vi "GUI_SmaractMCS.vi"() -> ()   [LabVIEW 2013]
uses:
  Shared/GUI_Template/GUI_master/tcp_new_data_event.ctl
  Shared/GUI_Template/GUI_master/tcp new data cluster.ctl
panel:
  in  "GUIdevice 1":string
  in  "Tab Control":enum32{"All Channels", "Internal"}(tab)
  in  "Home.Channel 3::1":enum16{"off", "on"}(ring) caption="Home.channel 3"
  in  "Home.Channel 2::1":enum16{"off", "on"}(ring) caption="Home.channel 2"
  in  "Position.Channel 3::1":dbl caption="Position.channel 3" min=0.0 max=10.0
  in  "Position.Channel 2::1":dbl caption="Position.channel 2" min=0.0 max=10.0
  in  "Position.Channel 1::1":dbl caption="Position.channel 1" min=0.0 max=10.0
  in  "Home.Channel 1::1":enum16{"off", "on"}(ring) caption="Home.channel 1"
  in  "localsavingpath::1":path caption="LocalSavingPath"
  out "tcp data event":T1
  in  "Refresh Button":bool
  out "device status::1":string="Initialized" caption="Status"
  in  "STOP":bool
  # "DAQ PAD USER INTERFACE"
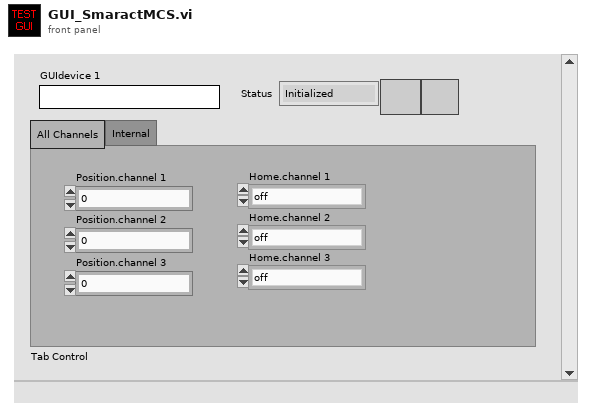
[diagram p1: front panel]
types:
  T1 = typedef "tcp_new_data_event.ctl" = refnum<user-event>
  T2 = enum32{"invalid app kind", "Development System", "Run Time System", "Student Edition", "Embedded LabVIEW", "Evaluation", "Custom"}
  T3 = typedef "tcp new data cluster.ctl" = cluster{"EventEnum":enum16{"new data", "connection status update"}, "Device name":string}
  T4 = enum32{"Invalid", "Standard", "Closed", "Hidden", "Minimized", "Maximized"}
  T5 = cluster{"Core":cluster{"Current VI Reference":refnum<vi>, "Close Panel on Exit?":bool}, "Your Boolean data":bool, "Your string data":string, "SuperGUI":cluster{"STOP queue":refnum<queue>, "SuperGUI ref":refnum<vi>}}
  T6 = cluster{"STOP queue":refnum<queue>, "SuperGUI ref":refnum<vi>}
  T7 = cluster{"Current VI Reference":refnum<vi>, "Close Panel on Exit?":bool}
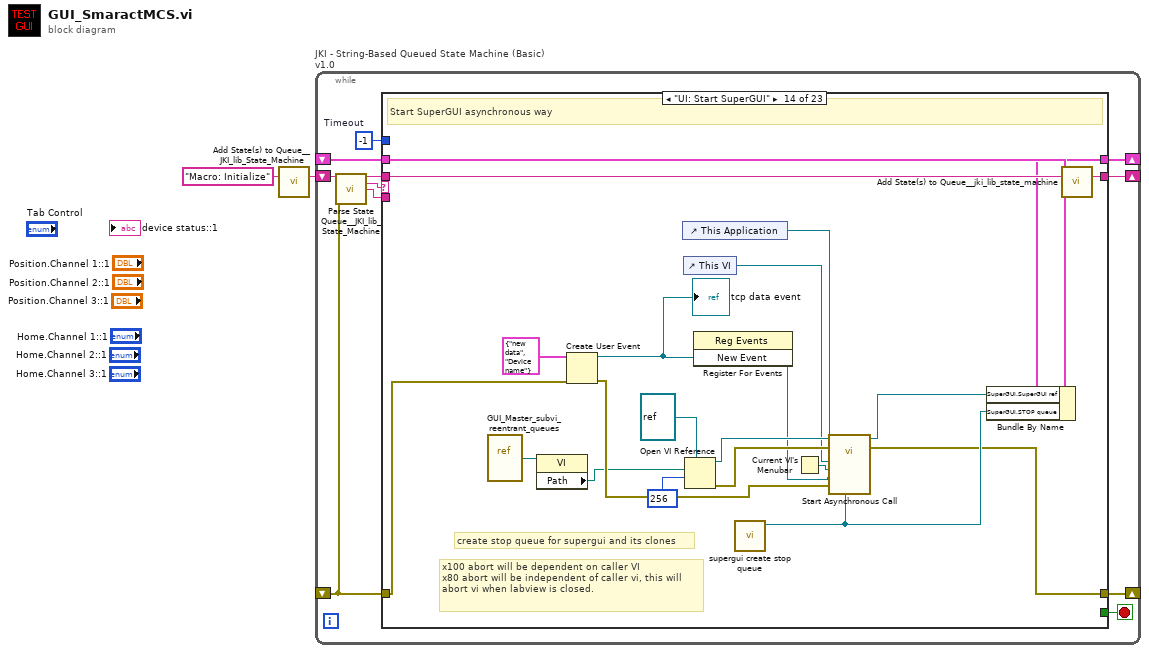
[diagram p0: block diagram]
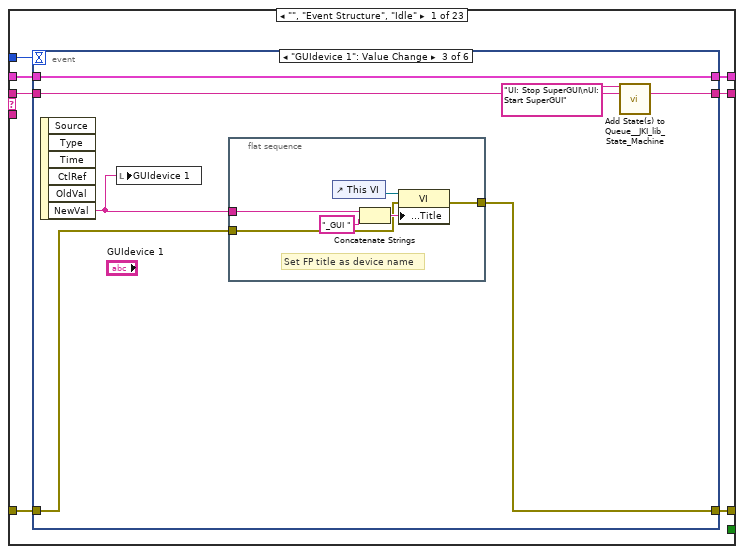
[diagram p2: hidden frame]
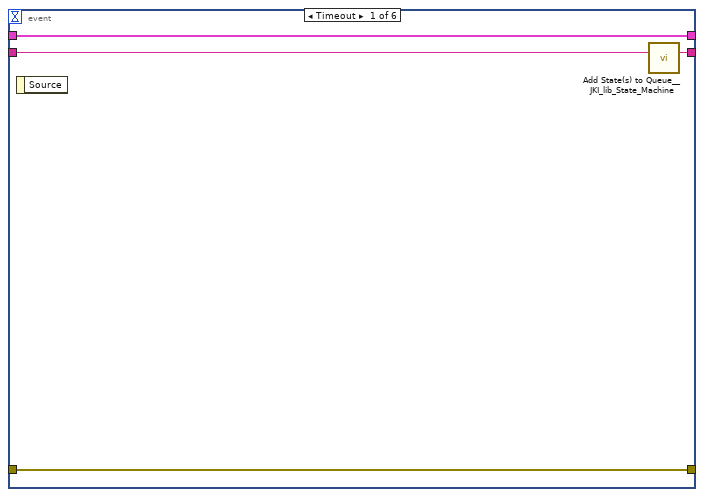
[diagram p3: hidden frame]
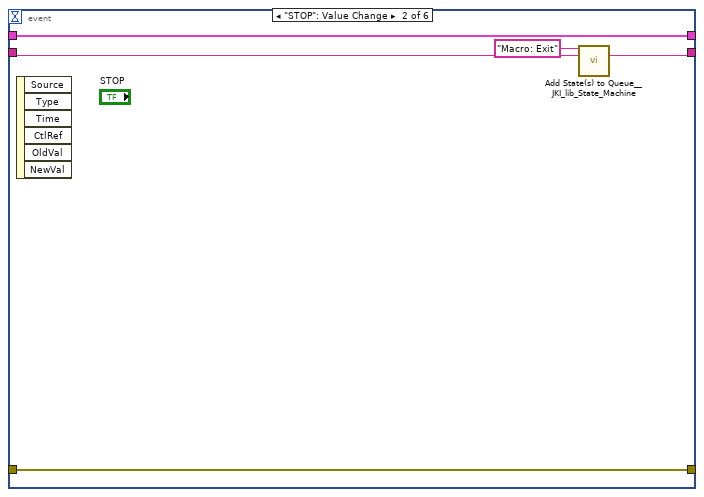
[diagram p4: hidden frame]
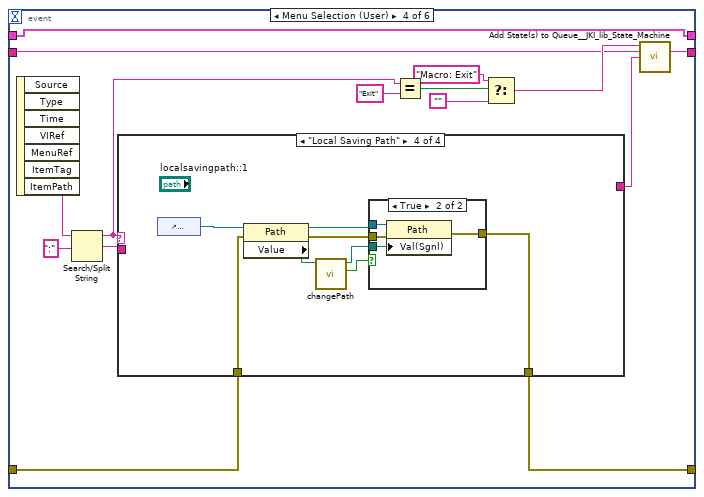
[diagram p5: hidden frame]
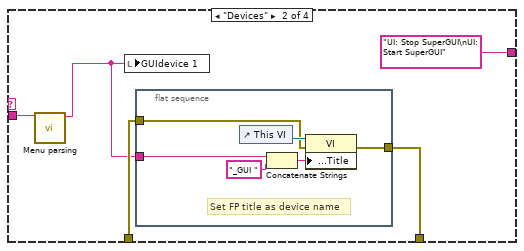
[diagram p7: hidden frame]
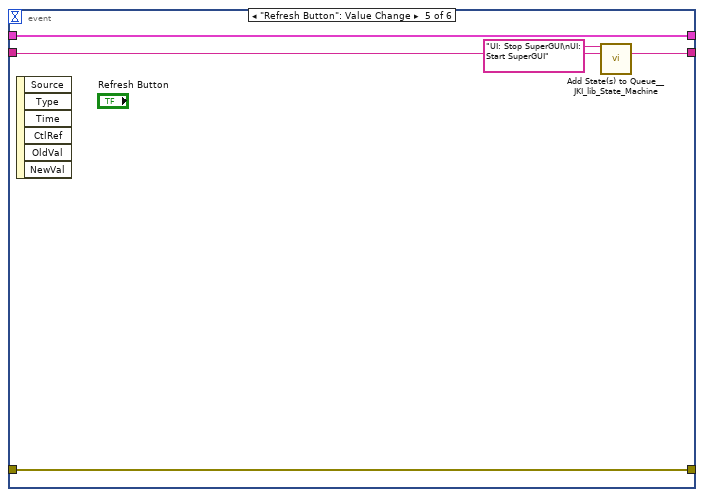
[diagram p10: hidden frame]
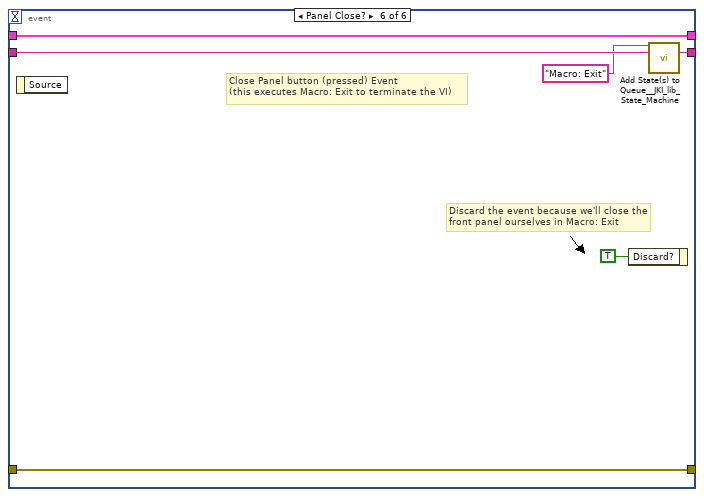
[diagram p11: hidden frame]
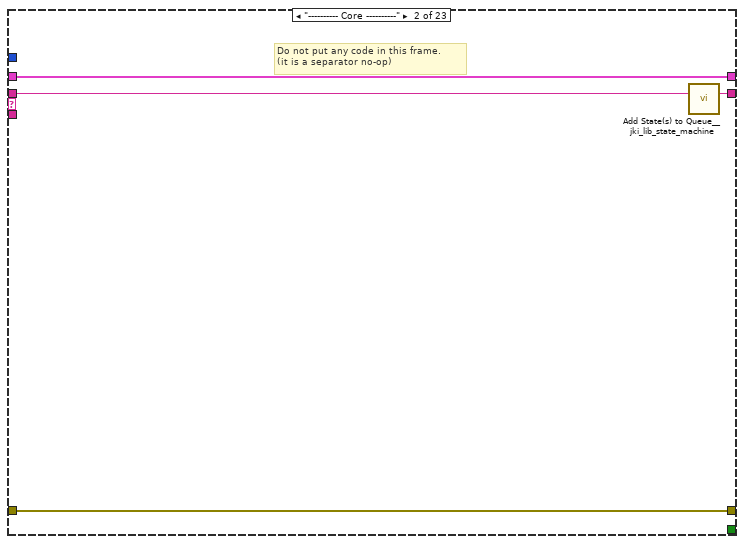
[diagram p12: hidden frame]
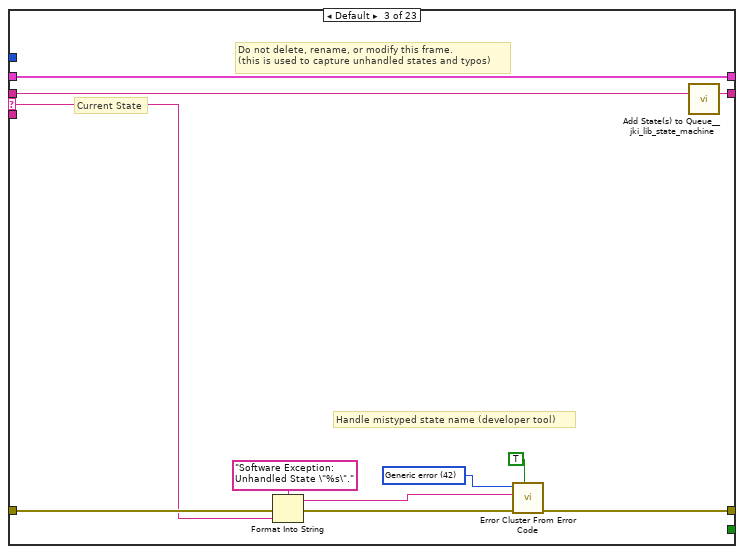
[diagram p13: hidden frame]
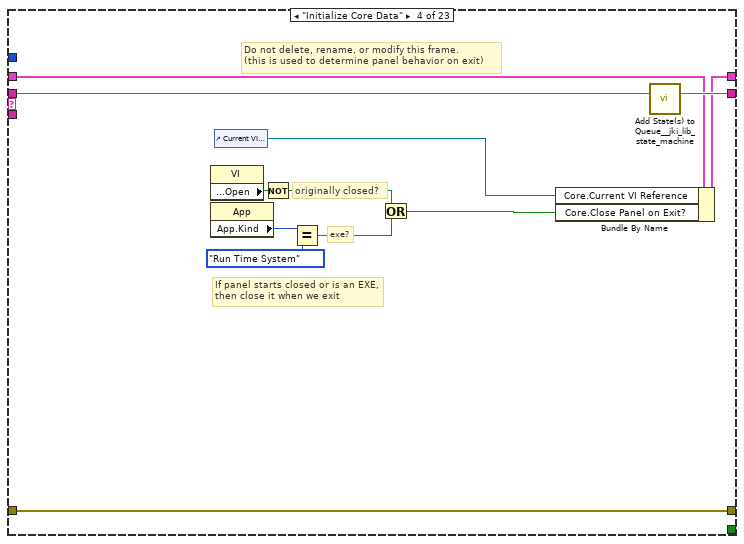
[diagram p14: hidden frame]
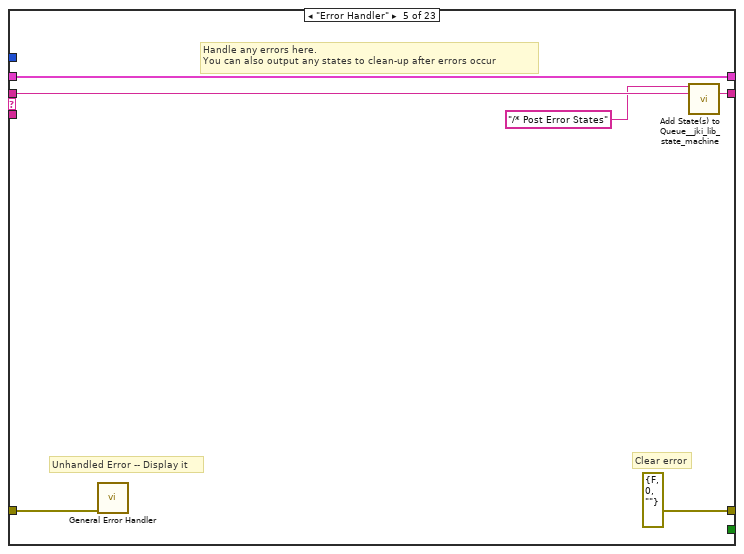
[diagram p15: hidden frame]
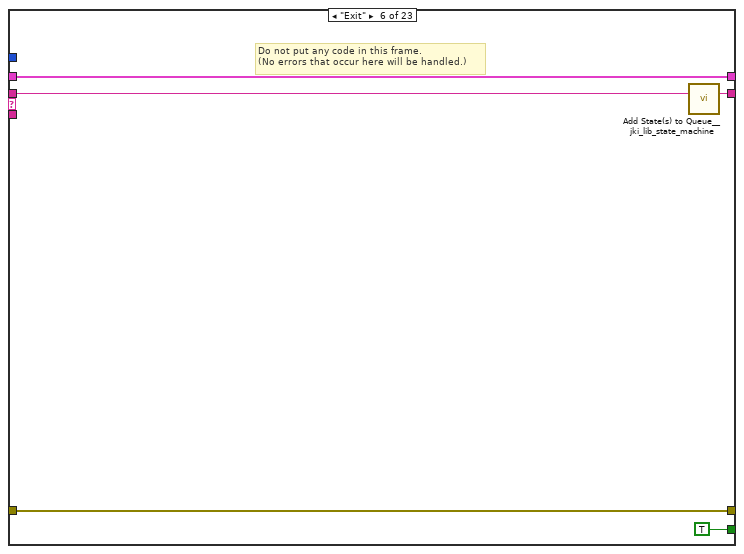
[diagram p16: hidden frame]
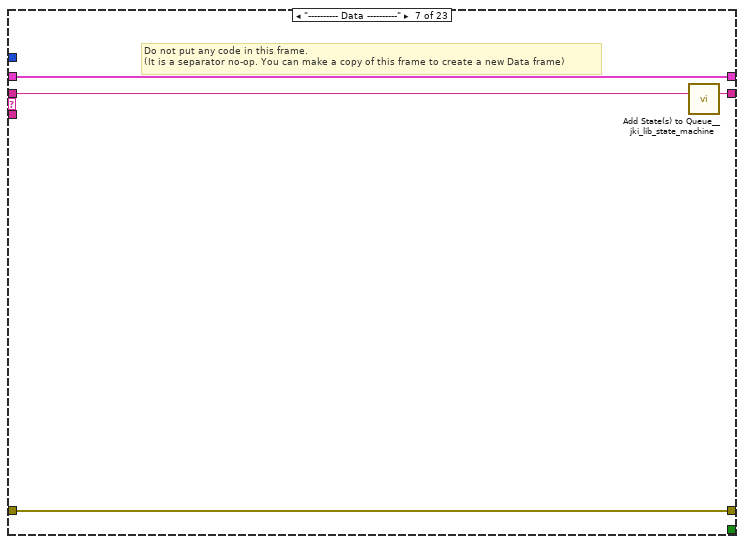
[diagram p17: hidden frame]
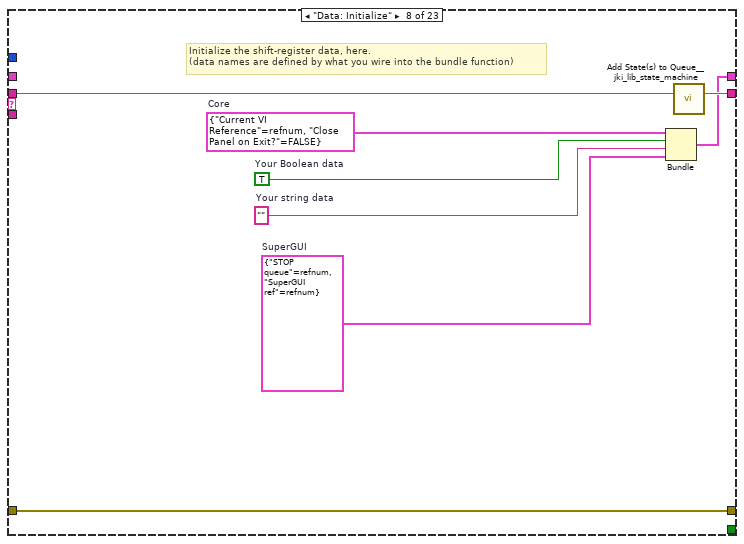
[diagram p18: hidden frame]
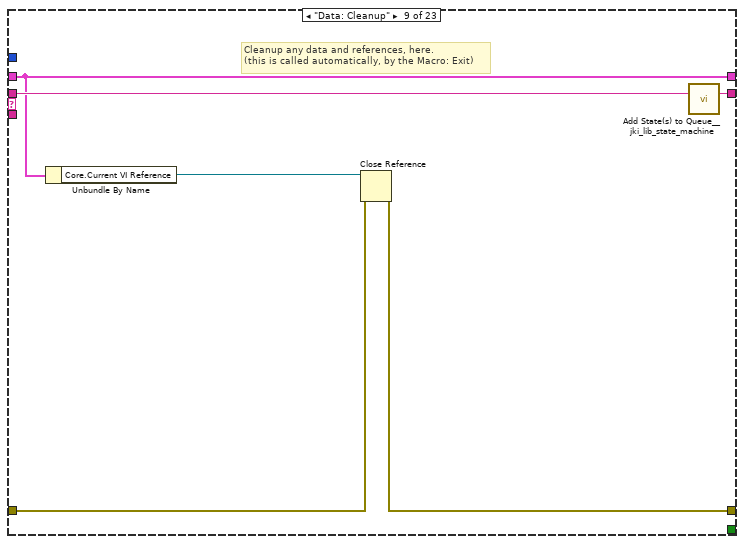
[diagram p19: hidden frame]
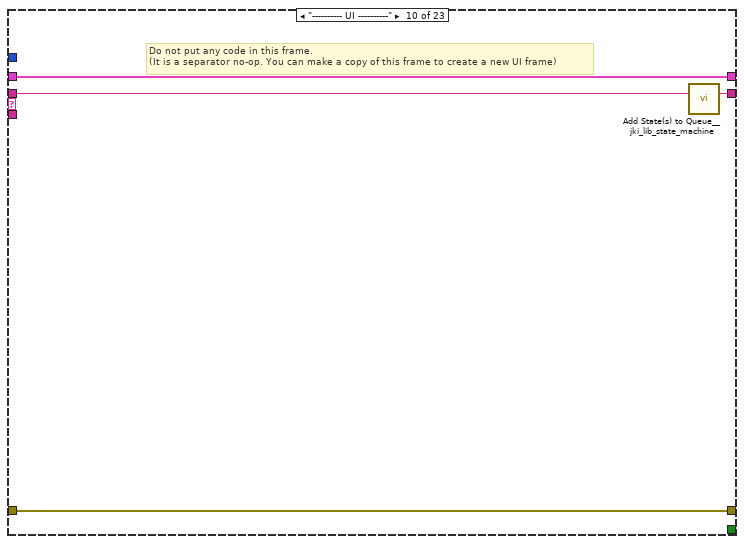
[diagram p20: hidden frame]
diagram:
  n1 = call <vilib>:"Add State(s) to Queue__JKI_lib_State_Machine.vi"("State(s) in (\"\")"="Macro: Initialize") -> ("States Out"=w2:string)  [unwired: 14 in]
  n2 = while "JKI - String-Based Queued State Machine (Basic) v1.0" {
    shift-right: [w6] -> _
    shift-left: _ -> [w5]
    shift-right: [w9] -> _
    shift-left: _ -> [w3]
    shift-right: [w8] -> _
    shift-left: w2 -> [w10]
    stop <- w7 stop-if-true
    w4 = -1  # Timeout
    n3 = call <vilib>:"Parse State Queue__JKI_lib_State_Machine.vi"("State Queue"=w10, "Error In (no error)"=w3) -> ("Remaining States"=w12:string, "Current State"=w13:string, "Arguments"=w11:string)  [unwired: 11 in]
    n4 = case shown="\"UI: Start SuperGUI\"" w13 {
      selector: w13 -> [_ _ w99 _ _ _ _ _ _ _ _ _ _ _ _ _ _ _ _ _ _ _ _]
      tunnel: w12 -> [w20 w98 w103 w121 w127 w132 w136 w144 w150 w154 w158 w166 w198 w232 w240 w246 w257 w283 w288 w298 w302 w306 w310]
      tunnel: w11 -> [_ _ _ _ _ _ _ _ _ _ _ _ _ _ _ w241 w251 _ _ _ _ _ _]
      tunnel: w5 -> [w18 w95 w101 w112 w124 w130 w133 _ w145 w151 w156 w164 w196 w223 w235 w244 w253 w280 w285 w295 w299 w303 w307]
      tunnel: [w17 w96 w105 w118 errorcluster {"status"=FALSE, "code"=0, "source"=""} ("error out") w129 w134 w141 w146 w152 w155 w161 w193 w216 w233 w242 w254 w281 w286 w296 w300 w304 w308] -> w9
      tunnel: w3 -> [w16 w96 w104 w118 w123 w129 w134 w141 w147 w152 w155 w163 w194 w217 w234 w243 w255 w281 w286 w296 w300 w304 w308]
      tunnel: [w19 w97 w102 w120 w126 w131 w135 w143 w149 w153 w157 w165 w197 w231 w239 w245 w256 w282 w287 w297 w301 w305 w309] -> w8
      tunnel: [_ _ _ _ _ TRUE _ _ _ _ _ _ _ _ _ _ _ _ _ _ _ _ _] -> w7
      tunnel: [w15 w95 w101 w119 w124 w130 w133 w142 w145 w151 w156 w164 w196 w222 w235 w244 w253 w280 w285 w295 w299 w303 w307] -> w6
      tunnel: w4 -> [w14 _ _ _ _ _ _ _ _ _ _ _ _ _ _ _ _ _ _ _ _ _ _]
      frame "", "Event Structure", "Idle" {
        n5 = event shown="[2] \"GUIdevice 1\": Value Change" {
          selector: _ -> [_ _ _ _ _ _]
          dyn-events: _ -> [_ _ _ _ _ _]
          timeout: w14 -> [_ _ _ _ _ _]
          tunnel: w20 -> [w24 w27 w33 w51 w86 w94]
          tunnel: [w23 w26 w32 w50 w85 w93] -> w19
          tunnel: w18 -> [w21 w29 w36 w57 w88 w91]
          tunnel: [w22 w28 w34 w44 w87 w92] -> w17
          tunnel: w16 -> [w22 w28 w35 w45 w87 w92]
          tunnel: [w21 w29 w36 w57 w88 w91] -> w15
          event Timeout {
            n6 = event-data() -> ()  [unwired: 1 in, 1 out]
            n7 = call <vilib>:"Add State(s) to Queue__JKI_lib_State_Machine.vi"("State(s) in (\"\")"=w24) -> ("States Out"=w23:string)  [unwired: 14 in]
          }
          event "STOP": Value Change {
            n8 = event-data() -> ()  [unwired: 1 in, 6 out]
            n9 = call <vilib>:"Add State(s) to Queue__JKI_lib_State_Machine.vi"("State(s) in Front (\"\")"="Macro: Exit", "State(s) in (\"\")"=w27) -> ("States Out"=w26:string)  [unwired: 13 in]
          }
          event "GUIdevice 1": Value Change {
            n10 = event-data() -> ("NewVal"=w30:string)  [unwired: 1 in, 5 out]
            n11 = local write "GUIdevice 1"(w30) -> ()
            n12 = flat-sequence {
              tunnel: [w39] -> w34
              tunnel: w35 -> [w38]
              tunnel: w30 -> [w37]
              frame #0 {
                # "Set FP title as device name"
                n13 = control-ref of="This VI"() -> (w42:refnum<vi>)
                n14 = Concatenate Strings(w37, "_GUI ") -> (w41:string)
                n15 = property class="VI"(reference=w42, error in=w38, "Front Panel.Title"=w41) -> (error out=w39:errorcluster)  [unwired: 1 out]
              }
            }
            n16 = call <vilib>:"Add State(s) to Queue__JKI_lib_State_Machine.vi"("State(s) in Front (\"\")"="UI: Stop SuperGUI\nUI: Start SuperGUI", "State(s) in (\"\")"=w33) -> ("States Out"=w32:string)  [unwired: 13 in]
          }
          event Menu Selection (User) {
            n17 = event-data() -> ("ItemPath"=w47:string)  [unwired: 1 in, 6 out]
            n18 = Search/Split String(string=w47, search string/char (-)=":") -> (substring before match=w43:string, match + rest of string=w46:string)  [unwired: 1 in, 1 out]
            n19 = case shown="\"Local Saving Path\"" w43 {
              tunnel: w46 -> [_ w63 _ _]
              tunnel: w45 -> [w58 w62 w70 w73]
              tunnel: [w58 w61 w70 w72] -> w44
              tunnel: [_ "UI: Stop SuperGUI\nUI: Start SuperGUI" _ _] -> w49
              frame "", Default {
              }
              frame "Devices" {
                n20 = call "Menu parsing.vi"("ItemPath"=w63) -> ("ItemPath"=w59:string)  [unwired: 9 in, 1 out]
                n21 = local write "GUIdevice 1"(w59) -> ()
                n22 = flat-sequence {
                  tunnel: [w66] -> w61
                  tunnel: w62 -> [w65]
                  tunnel: w59 -> [w64]
                  frame #0 {
                    # "Set FP title as device name"
                    n23 = control-ref of="This VI"() -> (w69:refnum<vi>)
                    n24 = Concatenate Strings(w64, "_GUI ") -> (w68:string)
                    n25 = property class="VI"(reference=w69, error in=w65, "Front Panel.Title"=w68) -> (error out=w66:errorcluster)  [unwired: 1 out]
                  }
                }
              }
              frame "Exit" {
              }
              frame "Local Saving Path" {
                n26 = control-ref of="localsavingpath::1"() -> (w74:refnum<vi>)
                n27 = property class="Path"(reference=w74, error in=w73) -> (reference out=w76:refnum<vi>, error out=w71:errorcluster, "Value"=w75:path)
                n28 = call "changePath.vi"("Local Saving in (h)"=w75) -> ("change (h)"=w77:bool, "Local Saving out (h)"=w78:path)  [unwired: 9 in]
                n29 = case shown="True" w77 {
                  tunnel: w76 -> [_ w83]
                  tunnel: w78 -> [_ w82]
                  tunnel: [w79 w81] -> w72
                  tunnel: w71 -> [w79 w80]
                  frame False {
                  }
                  frame True {
                    n30 = property class="Path"(reference=w83, error in=w80, "Val(Sgnl)"=w82) -> (error out=w81:errorcluster)  [unwired: 1 out]
                  }
                }
              }
            }
            n31 = Equal?(x=w43, y="Exit") -> (x = y?=w55:bool)
            n32 = Select(t="Macro: Exit", s=w55, f="") -> (s? t:f=w52:string)
            n33 = call <vilib>:"Add State(s) to Queue__JKI_lib_State_Machine.vi"("State(s) in Front (\"\")"=w52, "State(s) in (\"\")"=w51, "State(s) at Back (\"\")"=w49) -> ("States Out"=w50:string)  [unwired: 12 in]
          }
          event "Refresh Button": Value Change {
            n34 = event-data() -> ()  [unwired: 1 in, 6 out]
            n35 = call <vilib>:"Add State(s) to Queue__JKI_lib_State_Machine.vi"("State(s) in Front (\"\")"="UI: Stop SuperGUI\nUI: Start SuperGUI", "State(s) in (\"\")"=w86) -> ("States Out"=w85:string)  [unwired: 13 in]
          }
          event Panel Close? {
            # "Discard the event because we'll close the front panel ourselves in Macro: Exit"
            # "Close Panel button (pressed) Event\n(this executes Macro: Exit to terminate the VI)"
            n36 = event-data() -> ()  [unwired: 1 in, 1 out]
            n37 = event-data("Discard?"=TRUE) -> ()  [unwired: 1 in, 1 out]
            n38 = call <vilib>:"Add State(s) to Queue__JKI_lib_State_Machine.vi"("State(s) in Front (\"\")"="Macro: Exit", "State(s) in (\"\")"=w94) -> ("States Out"=w93:string)  [unwired: 13 in]
          }
        }
      }
      frame "---------- Core ----------" {
        # "Do not put any code in this frame.\n(it is a separator no-op)"
        n39 = call <vilib>:"Add State(s) to Queue__jki_lib_state_machine.vi"("State(s) in (\"\")"=w98) -> ("States Out"=w97:string)  [unwired: 14 in]
      }
      frame Default {
        w108 = 42 items=["No error", "Argument error", "Memory is full", "Out of zone", "End of file", "File already open", "Generic file I/O error", "File not found", "File permission error", "Disk is full", "Duplicate path", "Too many files open", "System feature not enabled", "Resource file not found", "Cannot add resource", "Resource not found", "Image not found", "Image memory error", "Pen does not exist", "Config type invalid", "Config token not found", "Config parse error", "Config memory error", "Bad external code format", "Bad external code offset", "External code not present", "Null window", "Destroy window error", "Null menu", "Print aborted", "Bad print record", "Print driver error", "Windows error during printing", "Memory error during printing", "Print dialog error", "Generic print error", "Invalid device refnum", "Device not found", "Device parameter error", "Device unit error", "Cannot open device", "Device call aborted", "Generic error", "Cancelled by user", "Object ID too low", "Object ID too high", "Object not in heap", "Unknown heap", "Unknown object (invalid DefProc)", "Unknown object (DefProc not in table)", "Message out of range", "Invalid (null) method", "Unknown message", "Manager call not supported", "Bad address", "Network operation in progress", "Network operation timed out", "Connection is busy", "Network attribute not supported", "Network error", "Address in use", "System out of memory", "Connection aborted", "Connection refused", "Not connected", "Already connected", "Connection closed", "Initialization error (interapplication manager)", "Bad occurrence", "Wait on unbound occurrence handler", "Occurrence queue overflow", "Datalog type conflict", "Unused", "Unrecognized type (interapplication manager)", "Memory corrupt", "Failed to make temporary DLL", "Old CIN version", "Drag socket not found", "Failed to load drop-object", "Failed to register OLE object", "Failed to release OLE object", "Format specifier type mismatch", "Unknown format specifier", "Too few format specifiers", "Too many format specifiers", "Scan failed", "Newer CIN version", "Error converting to variant", "Runtime menu error", "Password tampered", "Variant attribute not found", "Incompatible variant data type", "Event data is not available", "Event Store is not present", "Occurrence is not found", "Event Queue is not created", "Event info is not available", "Refnum passed is NULL", "Error retrieving Class GUID", "Error retrieving CoClass GUID", "Error retrieving TypeLib GUID.", "Bad built application magic bytes.", "Specific driver is different from the specific driver associated with the Logical Name.", "There is no session opened to the class driver.", "Max Error", "MAX - Error with config objects", "MAX - Error loading configuration", "MAX - Group not supported"]
        # "Current State"
        # "Do not delete, rename, or modify this frame.\n(this is used to capture unhandled states and typos)"
        # "Handle mistyped state name (developer tool)"
        n40 = Format Into String(format string="Software Exception: Unhandled State \"%s\"." ("message"), error in=w104, w99) -> (resulting string=w107:string, error out=w106:errorcluster)  [unwired: 1 in]
        n41 = call <vilib>:"Error Cluster From Error Code.vi"("show call chain? (False)"=TRUE, "error in (no error)"=w106, "error message (\"\")"=w107, "error code (0)"=w108) -> ("error out"=w105:errorcluster)  [unwired: 5 in]
        n42 = call <vilib>:"Add State(s) to Queue__jki_lib_state_machine.vi"("State(s) in (\"\")"=w103) -> ("States Out"=w102:string)  [unwired: 14 in]
      }
      frame "Initialize Core Data" {
        # "Do not delete, rename, or modify this frame.\n(this is used to determine panel behavior on exit)"
        # "originally closed?"
        # "exe?"
        # "If panel starts closed or is an EXE, then close it when we exit"
        n43 = property class="VI"() -> ("Front Panel.Open"=w117:bool)  [unwired: 2 in, 2 out]
        n44 = property class="App"() -> ("App.Kind"=w116:T2)  [unwired: 2 in, 2 out]
        n45 = control-ref of="Current VI Reference"() -> (w110:refnum<vi>)
        n46 = Not(x=w117) -> (.not. x?=w114:bool)
        n47 = Equal?(x=w116, y=T2."Run Time System" ("Application:Kind")) -> (x = y?=w113:bool)
        n48 = Or(x=w114, y=w113) -> (x .or. y?=w111:bool)
        n49 = Bundle By Name(cluster=w112, "Core.Current VI Reference"=w110, "Core.Close Panel on Exit?"=w111) -> (w119:T5)
        n50 = call <vilib>:"Add State(s) to Queue__jki_lib_state_machine.vi"("State(s) in (\"\")"=w121) -> ("States Out"=w120:string)  [unwired: 14 in]
      }
      frame "Error Handler" {
        # "Unhandled Error -- Display it"
        # "Handle any errors here.\nYou can also output any states to clean-up after errors occur"
        # "Clear error"
        n51 = call <vilib>:"General Error Handler.vi"("error in (no error)"=w123) -> ()  [unwired: 10 in, 5 out]
        n52 = call <vilib>:"Add State(s) to Queue__jki_lib_state_machine.vi"("State(s) in Front (\"\")"="/* Post Error States", "State(s) in (\"\")"=w127) -> ("States Out"=w126:string)  [unwired: 13 in]
      }
      frame "Exit" {
        # "Do not put any code in this frame.\n(No errors that occur here will be handled.)"
        n53 = call <vilib>:"Add State(s) to Queue__jki_lib_state_machine.vi"("State(s) in (\"\")"=w132) -> ("States Out"=w131:string)  [unwired: 14 in]
      }
      frame "---------- Data ----------" {
        # "Do not put any code in this frame.\n(It is a separator no-op. You can make a copy of this frame to create a new Data frame)"
        n54 = call <vilib>:"Add State(s) to Queue__jki_lib_state_machine.vi"("State(s) in (\"\")"=w136) -> ("States Out"=w135:string)  [unwired: 14 in]
      }
      frame "Data: Initialize" {
        w137 = T6 {"STOP queue"=refnum, "SuperGUI ref"=refnum}  # SuperGUI
        w138 = T7 {"Current VI Reference"=refnum, "Close Panel on Exit?"=FALSE}  # Core
        w140 = TRUE  # Your Boolean data
        w139 = ""  # Your string data
        # "Initialize the shift-register data, here.\n(data names are defined by what you wire into the bundle function)"
        n55 = Bundle("Core"=w138, "Your Boolean data"=w140, "Your string data"=w139, "SuperGUI"=w137) -> (w142:T5)  [unwired: 1 in]
        n56 = call <vilib>:"Add State(s) to Queue__jki_lib_state_machine.vi"("State(s) in (\"\")"=w144) -> ("States Out"=w143:string)  [unwired: 14 in]
      }
      frame "Data: Cleanup" {
        # "Cleanup any data and references, here.\n(this is called automatically, by the Macro: Exit)"
        n57 = Unbundle By Name(w145) -> ("Core.Current VI Reference"=w148:refnum<vi>)
        n58 = Close Reference(reference=w148, error in (no error)=w147) -> (error out=w146:errorcluster)
        n59 = call <vilib>:"Add State(s) to Queue__jki_lib_state_machine.vi"("State(s) in (\"\")"=w150) -> ("States Out"=w149:string)  [unwired: 14 in]
      }
      frame "---------- UI ----------" {
        # "Do not put any code in this frame.\n(It is a separator no-op. You can make a copy of this frame to create a new UI frame)"
        n60 = call <vilib>:"Add State(s) to Queue__jki_lib_state_machine.vi"("State(s) in (\"\")"=w154) -> ("States Out"=w153:string)  [unwired: 14 in]
      }
      frame "UI: Initialize" {
        # "Initialize the User Interface, here.\n(this is called automatically, by the Macro: Init)"
        n61 = call <vilib>:"Add State(s) to Queue__jki_lib_state_machine.vi"("State(s) in (\"\")"=w158) -> ("States Out"=w157:string)  [unwired: 14 in]
      }
      frame "UI: Update Device List" {
        n62 = call "getDevices.vi"("Device Class"="Smaract_MCS") -> ("All Devices"=w159:string[])
        n63 = Empty Array?(array=w159) -> (empty?=w160:bool)
        n64 = case shown="False" w160 {
          tunnel: w163 -> [w169 w192]
          tunnel: [w168 w192] -> w161
          tunnel: w159 -> [w167 _]
          frame False {
            n65 = Current VI's Menubar() -> (w172:refnum<k9>)
            n66 = Get Menu Item Info(7:"Devices" ("item tag"), 8:w169, 11:w172) -> (0:w178:errorcluster, 3:w174:refnum<k9>)  [unwired: 5 out]
            n67 = Set Menu Item Info(7:"Devices" ("item tag"), 8:w178, 9:TRUE ("enabled"), 11:w174) -> (0:w177:errorcluster, 3:w176:refnum<k9>)  [unwired: 3 in]
            n68 = First Call?() -> (First Call?: T/F=w170:bool)
            n69 = case shown="True" w170 {
              tunnel: w176 -> [_ w184]
              tunnel: w167 -> [_ w183]
              tunnel: w177 -> [w179 w181]
              tunnel: [w179 w180] -> w168
              frame False {
              }
              frame True {
                n70 = for {
                  tunnel: [w191] -> w185
                  tunnel: w183 -> [w189] mode=indexing
                  tunnel: w184 -> [w188]
                  tunnel: [w187] -> w182
                  tunnel: w181 -> [w186]
                  n71 = Insert Menu Items(5:"Devices" ("menu tag"), 6:w186, 7:w189, 8:w189, 9:w188) -> (0:w187:errorcluster, 3:w191:refnum<k9>)  [unwired: 1 in, 1 out]
                }
                n72 = Enable Menu Tracking(2:w182, 4:w185) -> (0:w180:errorcluster)  [unwired: 1 in, 1 out]
              }
            }
          }
          frame True {
          }
        }
        n73 = call <vilib>:"Add State(s) to Queue__jki_lib_state_machine.vi"("State(s) in (\"\")"=w166) -> ("States Out"=w165:string)  [unwired: 14 in]
      }
      frame "UI: Get Device Name" {
        n74 = First Call?() -> (First Call?: T/F=w195:bool)
        n75 = case shown="True" w195 {
          tunnel: w194 -> [w199 w201]
          tunnel: [w199 w200] -> w193
          frame False {
          }
          frame True {
            n76 = disable-structure "Get Device name from control for vi mode\nand command line arg for exe" shown="RUN_TIME_ENGINE==True" {
              disable-tunnel: w201 -> [_ w203]
              disable-tunnel: [_ w202] -> w200
              frame condition #0 (active) {
              }
              frame condition #1 {
                n77 = control-ref of="This Application"() -> (w211:refnum<vi>)
                n78 = property class="App"(reference=w211) -> ("App.Args"=w210:string[])  [unwired: 1 in, 2 out]
                n79 = Index Array(array=w210, index #1=1 ("index")) -> (element #1=w204:string)  [unwired: 2 in, 2 out]
                n80 = Empty String/Path?(string/path=w204) -> (empty?=w208:bool)
                n81 = control-ref of="This VI"() -> (w207:refnum<vi>)
                n82 = case shown="False" w208 {
                  tunnel: w204 -> [w212 _]
                  frame False {
                    n83 = local write "GUIdevice 1"(w212) -> ()
                  }
                  frame True {
                  }
                }
                n84 = Concatenate Strings(w204, "_GUI ") -> (w206:string)
                n85 = property class="VI"(reference=w207, error in=w203, "Front Panel.Title"=w206) -> (error out=w202:errorcluster)  [unwired: 1 out]
              }
            }
          }
        }
        n86 = call <vilib>:"Add State(s) to Queue__jki_lib_state_machine.vi"("State(s) in (\"\")"=w198) -> ("States Out"=w197:string)  [unwired: 14 in]
      }
      frame "UI: Start SuperGUI" {
        # "create stop queue for supergui and its clones"
        # "x100 abort will be dependent on caller VI\nx80 abort will be independent of caller vi, this will abort vi when labview is closed."
        # "Start SuperGUI asynchronous way"
        n87 = vi-ref "GUI_Master_subvi_reentrant_queues.vi"() -> (w215:refnum<vi>)
        n88 = property class="VI"(reference=w215) -> ("Path"=w214:path)  [unwired: 1 in, 2 out]
        n89 = Create User Event(user event datatype=T3 {"EventEnum"=enum."new data", "Device name"="Device name"} ("New Event"), error in=w217) -> (user event=w218:refnum<user-event>, error out=w224:errorcluster)
        "tcp data event" <- w218
        n90 = control-ref of="This Application"() -> (w221:refnum<vi>)
        n91 = control-ref of="This VI"() -> (w220:refnum<vi>)
        n92 = Open VI Reference(type specifier VI Refnum (for type only)=refnum<vi> refnum, vi path=w214, options=256) -> (vi reference=w230:refnum<vi>, error out=w229:errorcluster)  [unwired: 3 in]
        n93 = register-events(w218) -> ()  [unwired: 2 in, 2 out]
        n94 = call "supergui create stop queue.vi"() -> ("STOP Queue out"=w226:refnum<queue>)  [unwired: 11 in]
        n95 = Current VI's Menubar() -> (w219:refnum<k9>)
        n96 = call-by-ref "Start Asynchronous Call"(reference=w230, error in=w229, "STOP Queue in"=w226, "This Application"=w221, 8:"error in (no error)"=w224, "tcp data event"=w218, "Caller menu reference"=w219, "Caller VI ref"=w220) -> (reference out=w213:refnum<vi>, error out=w216:errorcluster)  [unwired: 5 in, 1 out]
        n97 = Bundle By Name(cluster=w223, "SuperGUI.SuperGUI ref"=w213, "SuperGUI.STOP queue"=w226) -> (w222:T5)
        n98 = call <vilib>:"Add State(s) to Queue__jki_lib_state_machine.vi"("State(s) in (\"\")"=w232) -> ("States Out"=w231:string)  [unwired: 14 in]
      }
      frame "UI: Stop SuperGUI" {
        # "Stop Supergui Clone and wait until it exit properly"
        n99 = Unbundle By Name(w235) -> ("SuperGUI.SuperGUI ref"=w237:refnum<vi>, "SuperGUI.STOP queue"=w236:refnum<queue>)
        n100 = Release Queue(queue=w236, error in (no error)=w234) -> (error out=w238:errorcluster)  [unwired: 1 in, 2 out]
        n101 = call-by-ref "Wait On Asynchronous Call"(reference=w237, error in=w238) -> ("error out"=w233:errorcluster)  [unwired: 11 in, 2 out]
        n102 = call <vilib>:"Add State(s) to Queue__jki_lib_state_machine.vi"("State(s) in (\"\")"=w240) -> ("States Out"=w239:string)  [unwired: 14 in]
      }
      frame "UI: Cursor Set" {
        # "Argument"
        # "Set and Unset Cursor Busy.\n(Usage: \"UI: Cursor Set >> Busy|Idle\")"
        n103 = case shown="\"Idle\", Default" w241 {
          tunnel: w243 -> [w248 w250]
          tunnel: [w247 w249] -> w242
          frame "Idle", Default {
            n104 = call <vilib>:"Unset Busy.vi"("error in (no error)"=w248) -> ("error out"=w247:errorcluster)  [unwired: 10 in]
          }
          frame "Busy" {
            n105 = call <vilib>:"Set Busy.vi"("error in (no error)"=w250) -> ("error out"=w249:errorcluster)  [unwired: 9 in, 1 out]
          }
        }
        n106 = call <vilib>:"Add State(s) to Queue__jki_lib_state_machine.vi"("State(s) in (\"\")"=w246) -> ("States Out"=w245:string)  [unwired: 14 in]
      }
      frame "UI: Front Panel State" {
        # "Argument"
        # "Set Front Panel Open or Closed\n(Usage: \"UI: Front Panel State >> Open|Close\")"
        n107 = Unbundle By Name(w253) -> ("Core.Current VI Reference"=w252:refnum<vi>)
        n108 = case shown="\"Open\", Default" w251 {
          tunnel: w255 -> [w261 w274]
          tunnel: [w263 w275] -> w254
          tunnel: w252 -> [w262 w272]
          frame "Open", Default {
            n109 = property class="VI"(reference=w262, error in=w261) -> (reference out=w259:refnum<vi>, error out=w260:errorcluster, "Front Panel.Open"=w258:bool)
            n110 = case shown="False" w258 {
              tunnel: [w266 w269] -> w263
              tunnel: w260 -> [w265 w269]
              tunnel: w259 -> [w264 _]
              frame False {
                n111 = invoke class="VI" method="FP.Open"(reference=w264, error in=w265, "Activate"=TRUE, "State"=T4."Standard") -> (error out=w266:errorcluster)  [unwired: 1 in, 4 out]
              }
              frame True {
              }
            }
          }
          frame "Close" {
            n112 = property class="VI"(reference=w272, error in=w274) -> (reference out=w271:refnum<vi>, error out=w273:errorcluster, "Front Panel.Open"=w270:bool)
            n113 = case shown="True" w270 {
              tunnel: [w276 w279] -> w275
              tunnel: w273 -> [w276 w278]
              tunnel: w271 -> [_ w277]
              frame False {
              }
              frame True {
                n114 = invoke class="VI" method="FP.Close"(reference=w277, error in=w278) -> (error out=w279:errorcluster)  [unwired: 1 in, 2 out]
              }
            }
          }
        }
        n115 = call <vilib>:"Add State(s) to Queue__jki_lib_state_machine.vi"("State(s) in (\"\")"=w257) -> ("States Out"=w256:string)  [unwired: 14 in]
      }
      frame "---------- Macro ----------" {
        # "Do not put any code in this frame.\n(It is a separator no-op. You can make a copy of this frame to create a new Macro frame)"
        n116 = call <vilib>:"Add State(s) to Queue__jki_lib_state_machine.vi"("State(s) in (\"\")"=w283) -> ("States Out"=w282:string)  [unwired: 14 in]
      }
      frame "Macro: Initialize" {
        # "Initialization Macro\n(This is called once, when the VI starts)"
        n117 = call <vilib>:"Add State(s) to Queue__jki_lib_state_machine.vi"("State(s) in Front (\"\")"="Data: Initialize\nInitialize Core Data\nUI: Initialize\nUI: Update Device List\nUI: Get Device Name\nUI: Start SuperGUI\nUI: Front Panel State >> Open", "State(s) in (\"\")"=w288) -> ("States Out"=w287:string)  [unwired: 13 in]
      }
      frame "Macro: Exit" {
        # "Exit Macro\n(This is called once, when the VI exits)"
        n118 = Unbundle By Name(w295) -> ("Core.Close Panel on Exit?"=w294:bool)
        n119 = Select(t="UI: Front Panel State >> Close", s=w294, f="") -> (s? t:f=w291:string)
        n120 = call <vilib>:"Add State(s) to Queue__jki_lib_state_machine.vi"("State(s) in (\"\")"=w291, "State(s) at Back (\"\")"="Data: Cleanup\nExit") -> ("States Out"=w289:string)  [unwired: 13 in]
        n121 = call <vilib>:"Add State(s) to Queue__jki_lib_state_machine.vi"("State(s) in Front (\"\")"=w289, "State(s) in (\"\")"=w298) -> ("States Out"=w297:string)  [unwired: 13 in]
      }
      frame "---------- New Category ----------" {
        # "Template Separator\n(You can make a copy of, or modify, this frame)"
        n122 = call <vilib>:"Add State(s) to Queue__jki_lib_state_machine.vi"("State(s) in (\"\")"=w302) -> ("States Out"=w301:string)  [unwired: 14 in]
      }
      frame "New Category: 1" {
        # "Your code here.\n(You can make a copy of, or modify, this frame)"
        n123 = call <vilib>:"Add State(s) to Queue__jki_lib_state_machine.vi"("State(s) in (\"\")"=w306) -> ("States Out"=w305:string)  [unwired: 14 in]
      }
      frame "New Category: 2" {
        # "Your code here.\n(You can make a copy of, or modify, this frame)"
        n124 = call <vilib>:"Add State(s) to Queue__jki_lib_state_machine.vi"("State(s) in (\"\")"=w310) -> ("States Out"=w309:string)  [unwired: 14 in]
      }
    }
  }
